vi "Begin.vi"(8 "error in":errorcluster) -> (0 "error out":errorcluster)   [LabVIEW 2019]
doc: "Called before other user functions, this VI is expected to open initial I/O refnums, load in file data, and do all program initialization. Notice that the <B>error out</B> terminal is simply used for data flow. Wiring it to other structures or subVIs ensures that this VI runs first."
uses:
  <vilib>/Rock Robotics/WPI/SafetyOutput/WPI_SafetyOutputConfigMenu.ctl
  <vilib>/Rock Robotics/WPI/DriverStation/WPI_DriverStationRobotMode2.ctl
  <vilib>/Rock Robotics/WPI/Joystick/WPI_JoystickDeviceEnum.ctl
  <vilib>/Rock Robotics/WPI/ThirdParty/REV Robotics/SPARK MAX/Typedef/Spark MAX Idle Mode.ctl
  <vilib>/Rock Robotics/WPI/ThirdParty/REV Robotics/SPARK MAX/Typedef/Spark MAX Motor Type.ctl
  <vilib>/Rock Robotics/WPI/Solenoid/WPI_SolenoidChannel.ctl
  <vilib>/Rock Robotics/WPI/ThirdParty/Phoenix-LabVIEW/Motor Controller/Controls/CTRE_Phoenix_MotorControl_ControlMode.ctl
  <vilib>/Rock Robotics/SystemInterfaces/DIO/FPGA_DIOChannel.ctl
  <vilib>/Rock Robotics/WPI/Encoder/WPI_EncoderType.ctl
  Robot Global Data.vi
  <vilib>/Rock Robotics/Network Tables/NT Write String Array.vi
  <vilib>/Rock Robotics/WPI/RobotDrive/WPI_RobotDriveOpen2MotorWithExistingMotors.vi
  <vilib>/Rock Robotics/WPI/Solenoid/WPI_SolenoidOpenDouble.vi
  <vilib>/Rock Robotics/WPI/Counter/WPI_CounterDigitalInputToDigitalSource.vi
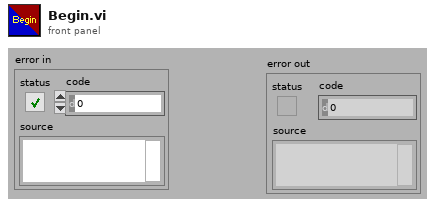
[diagram p1: front panel]
types:
  T1 = typedef "WPI_EncoderType.ctl" = enum16{"1x", "2x", "4x"}
  T2 = typedef "FPGA_DIOChannel.ctl" = enum8{"DIO 0", "DIO 1", "DIO 2", "DIO 3", "DIO 4", "DIO 5", "DIO 6", "DIO 7", "DIO 8", "DIO 9", "DIO MXP 0", "DIO MXP 1", "DIO MXP 2", "DIO MXP 3", "DIO MXP 4", "DIO MXP 5", "DIO MXP 6", "DIO MXP 7", "DIO MXP 8", "DIO MXP 9", "DIO MXP 10", "DIO MXP 11", "DIO MXP 12", "DIO MXP 13", "DIO MXP 14", "DIO MXP 15", "SPI Port CS1", "SPI Port CS2", "SPI Port CS3", "SPI Port MISO", "SPI Port MOSI", "Invalid"}
  T3 = typedef "CTRE_Phoenix_MotorControl_ControlMode.ctl" = u16
  T4 = typedef "WPI_SolenoidChannel.ctl" = enum8{"Solenoid 0", "Solenoid 1", "Solenoid 2", "Solenoid 3", "Solenoid 4", "Solenoid 5", "Solenoid 6", "Solenoid 7", "Invalid"}
  T5 = typedef "WPI_JoystickDeviceEnum.ctl" = enum16{"USB 0", "USB 1", "USB 2", "USB 3", "USB 4", "USB 5"}
  T6 = typedef "Spark MAX Motor Type.ctl" = enum16{"Brushed", "Brushless"}
  T7 = typedef "Spark MAX Idle Mode.ctl" = enum16{"Coast", "Brake"}
  T8 = typedef "WPI_DriverStationRobotMode2.ctl" = enum16{"Autonomous Disabled", "Autonomous Enabled", "Teleop Disabled", "Teleop Enabled", "Disconnected", "Finish", "Test Disabled", "Test Enabled", "Emergency Stopped"}
  T9 = typedef "WPI_SafetyOutputConfigMenu.ctl" = enum16{"Enable", "Disable"}
  T10 = typedef "WPI_MotorControlDeviceRef.ctl" = cluster{"DeviceStatus":errorcluster, "Type":T11, "PWM":cluster{"PWM Channel":T12, "DeadBand":T13}, "CAN":cluster{"Device Number":u8, "SetOutput VI Ref":variant, "GetOutput VI Ref":variant, "Enable VI Ref":variant, "Disable VI Ref":variant, "Data":variant}, "Invert":bool, "DIO PWM":cluster{"PWM \"Enable\" Channel":T12, "DIOChannel":T2, "PWM Rate":dbl}}
  T11 = typedef "WPI_MotorControlType.ctl" = enum16{"PWM", "CAN", "DIO PWM"}
  T12 = typedef "FPGA_DIOPWMChannel.ctl" = enum8{"PWM 0", "PWM 1", "PWM 2", "PWM 3", "PWM 4", "PWM 5", "PWM 6", "PWM 7", "PWM 8", "PWM 9", "PWM MXP 0", "PWM MXP 1", "PWM MXP 2", "PWM MXP 3", "PWM MXP 4", "PWM MXP 5", "PWM MXP 6", "PWM MXP 7", "PWM MXP 8", "PWM MXP 9", "Invalid"}
  T13 = typedef "WPI_PWMDeadband.ctl" = cluster{"Name":string, "maxPositivePwm":i32, "minPositivePwm":i32, "centerPwm":i32, "maxNegativePwm":i32, "minNegativePwm":i32, "angularRange":u16}
  T14 = typedef "WPI_RobotDriveDevRef.ctl" = cluster{"DevStatus":errorcluster, "Motors[]":T10[], "Square Inputs":bool, "Max Output":dbl}
  T15 = typedef "WPI_JoystickDevRef.ctl" = cluster{"Device":T5}
  T16 = typedef "WPI_SolenoidDevRef.ctl" = cluster{"DevStatus":errorcluster, "Pneumatics Control Module":u8, "Forward Solenoid Channel":T4, "Reverse Solenoid Channel":T4}
  T17 = typedef "WPI_DigitalInputDevRef.ctl" = cluster{"DevStatus":errorcluster, "DIO Channel":T2}
  T18 = typedef "FPGA_CounterEncoderSourceConvertionLVSourceType.ctl" = cluster{"DevStatus":errorcluster, "AnalogTriggerMode?":bool, "DigitalMode":cluster{"DIO Channel":T19}, "AnalogTriggerMode":cluster{"AnalogTriggerIndex":T20, "OutputType":T21}}
  T19 = typedef "FPGA_DIODigitalSourceChannel.ctl" = enum8{"DIO 0", "DIO 1", "DIO 2", "DIO 3", "DIO 4", "DIO 5", "DIO 6", "DIO 7", "DIO 8", "DIO 9", "DIO MXP 0", "DIO MXP 1", "DIO MXP 2", "DIO MXP 3", "DIO MXP 4", "DIO MXP 5", "DIO MXP 6", "DIO MXP 7", "DIO MXP 8", "DIO MXP 9", "DIO MXP 10", "DIO MXP 11", "DIO MXP 12", "DIO MXP 13", "DIO MXP 14", "DIO MXP 15", "SPI Port CS1", "SPI Port CS2", "SPI Port CS3", "SPI Port MISO", "SPI Port MOSI", "Disabled"}
  T20 = typedef "FPGA_AnalogTriggerIndex.ctl" = enum8{"Trig 0", "Trig 1", "Trig 2", "Trig 3", "Trig 4", "Trig 5", "Trig 6", "Trig 7", "Invalid"}
  T21 = typedef "FPGA_AnalogTriggerOutType.ctl" = enum16{"InWindow", "TriggerState", "Rising", "Falling"}
  T22 = typedef "WPI_EncoderDevRef.ctl" = cluster{"DevStatus":errorcluster, "EncoderIndex":T23, "CounterIndex":T24, "DistancePerCount":dbl, "Decoding Type":T1}
  T23 = typedef "FPGA_EncoderIdx.ctl" = enum8{"Enc 0", "Enc 1", "Enc 2", "Enc 3", "Enc 4", "Enc 5", "Enc 6", "Enc 7", "Invalid"}
  T24 = typedef "FPGA_CounterCtrSystemIndex.ctl" = enum8{"Ctr 0", "Ctr 1", "Ctr 2", "Ctr 3", "Ctr 4", "Ctr 5", "Ctr 6", "Ctr 7", "Invalid"}
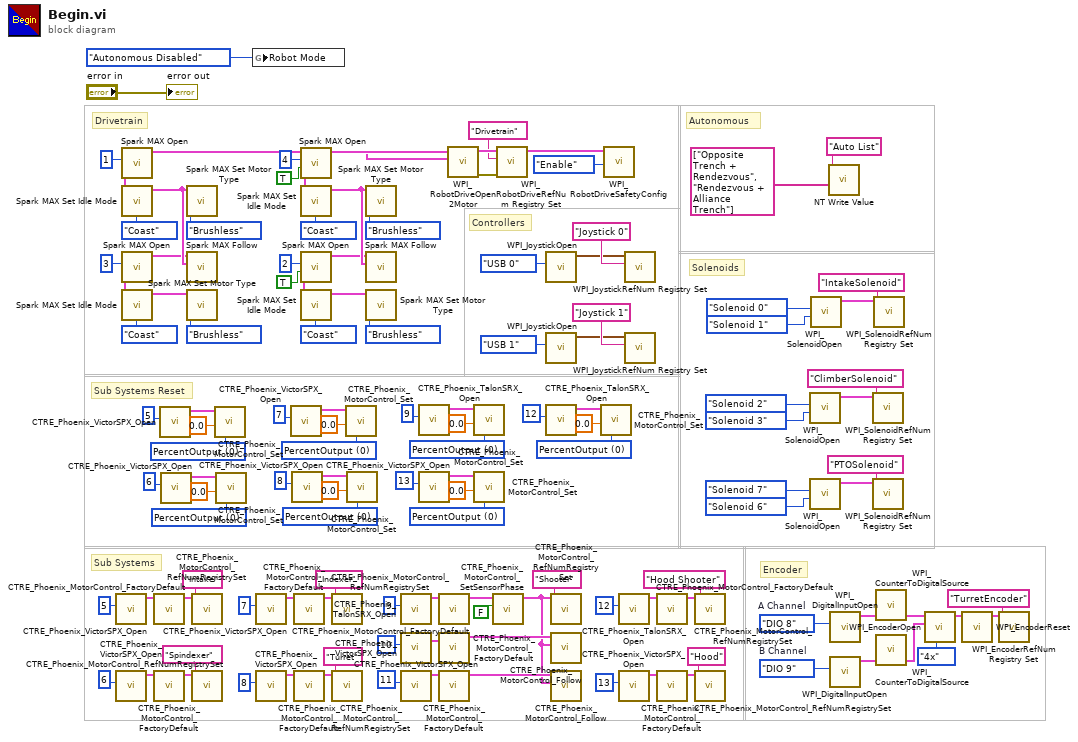
[diagram p0: block diagram]
diagram:
  w8 = FPGA_DIOChannel."DIO 9"  # B Channel
  w7 = FPGA_DIOChannel."DIO 8"  # A Channel
  w16 = T3 0 items=["PercentOutput"=0, "Position"=1, "Velocity"=2, "Current"=3, "Follower"=5, "MotionProfile"=6, "MotionMagic"=7, "MotionProfileArc"=10, "Disabled"=15] ("Control Mode")
  w19 = T3 0 items=["PercentOutput"=0, "Position"=1, "Velocity"=2, "Current"=3, "Follower"=5, "MotionProfile"=6, "MotionMagic"=7, "MotionProfileArc"=10, "Disabled"=15] ("Control Mode")
  w24 = T3 0 items=["PercentOutput"=0, "Position"=1, "Velocity"=2, "Current"=3, "Follower"=5, "MotionProfile"=6, "MotionMagic"=7, "MotionProfileArc"=10, "Disabled"=15] ("Control Mode")
  w32 = T3 0 items=["PercentOutput"=0, "Position"=1, "Velocity"=2, "Current"=3, "Follower"=5, "MotionProfile"=6, "MotionMagic"=7, "MotionProfileArc"=10, "Disabled"=15] ("Control Mode")
  w29 = T3 0 items=["PercentOutput"=0, "Position"=1, "Velocity"=2, "Current"=3, "Follower"=5, "MotionProfile"=6, "MotionMagic"=7, "MotionProfileArc"=10, "Disabled"=15] ("Control Mode")
  w37 = T3 0 items=["PercentOutput"=0, "Position"=1, "Velocity"=2, "Current"=3, "Follower"=5, "MotionProfile"=6, "MotionMagic"=7, "MotionProfileArc"=10, "Disabled"=15] ("Control Mode")
  w39 = T3 0 items=["PercentOutput"=0, "Position"=1, "Velocity"=2, "Current"=3, "Follower"=5, "MotionProfile"=6, "MotionMagic"=7, "MotionProfileArc"=10, "Disabled"=15] ("Control Mode")
  # "Encoder"
  # "Autonomous"
  # "Sub Systems Reset"
  # "Solenoids"
  # "Controllers"
  # "Sub Systems"
  # "Drivetrain"
  n1 = call <vilib>:"CTRE_Phoenix_VictorSPX_Open.vi"("Device Number"=u8 5) -> ("CAN Talon SRX Ref"=w62:T10)  [unwired: 9 in, 1 out]
  n2 = call <vilib>:"CTRE_Phoenix_VictorSPX_Open.vi"("Device Number"=u8 6) -> ("CAN Talon SRX Ref"=w64:T10)  [unwired: 9 in, 1 out]
  n3 = call <vilib>:"Spark MAX Open.vi"("Device Number"=u8 1) -> ("MotorControlDeviceRef"=w88:T10)  [unwired: 9 in, 1 out]
  n4 = call <vilib>:"Spark MAX Set Idle Mode.vi"("Idle Mode"=Spark_MAX_Idle_Mode."Coast", "MotorControlDeviceRef in"=w88) -> ("MotorControlDeviceRef out"=w104:T10)  [unwired: 8 in, 1 out]
  n5 = call <vilib>:"Spark MAX Open.vi"("Device Number"=u8 3) -> ("MotorControlDeviceRef"=w103:T10)  [unwired: 9 in, 1 out]
  n6 = call <vilib>:"Spark MAX Set Idle Mode.vi"("Idle Mode"=Spark_MAX_Idle_Mode."Coast", "MotorControlDeviceRef in"=w103) -> ("MotorControlDeviceRef out"=w108:T10)  [unwired: 8 in, 1 out]
  n7 = call <vilib>:"CTRE_Phoenix_MotorControl_FactoryDefault.vi"("PhoenixMotorControlDevRef"=w62) -> ("PhoenixMotorControlDevRef"=w63:T10)  [unwired: 9 in, 1 out]
  n8 = call <vilib>:"CTRE_Phoenix_MotorControl_FactoryDefault.vi"("PhoenixMotorControlDevRef"=w64) -> ("PhoenixMotorControlDevRef"=w65:T10)  [unwired: 9 in, 1 out]
  n9 = call <vilib>:"CTRE_Phoenix_VictorSPX_Open.vi"("Device Number"=u8 5) -> ("CAN Talon SRX Ref"=w36:T10)  [unwired: 9 in, 1 out]
  n10 = call <vilib>:"CTRE_Phoenix_VictorSPX_Open.vi"("Device Number"=u8 6) -> ("CAN Talon SRX Ref"=w40:T10)  [unwired: 9 in, 1 out]
  n11 = call <vilib>:"Spark MAX Set Motor Type.vi"("Motor Type"=Spark_MAX_Motor_Type."Brushless", "MotorControlDevRef"=w104) -> ()  [unwired: 8 in, 2 out]
  n12 = call <vilib>:"Spark MAX Follow.vi"("Master Controller"=w104, "MotorControlDeviceRef"=w103) -> ()  [unwired: 8 in, 2 out]
  n13 = call <vilib>:"Spark MAX Set Motor Type.vi"("Motor Type"=Spark_MAX_Motor_Type."Brushless", "MotorControlDevRef"=w108) -> ()  [unwired: 8 in, 2 out]
  n14 = call <vilib>:"CTRE_Phoenix_MotorControl_RefNumRegistrySet.vi"("refnum name"="Intake", "PhoenixMotorControlDevRef"=w63) -> ()  [unwired: 8 in, 2 out]
  n15 = call <vilib>:"CTRE_Phoenix_MotorControl_RefNumRegistrySet.vi"("refnum name"="Spindexer", "PhoenixMotorControlDevRef"=w65) -> ()  [unwired: 8 in, 2 out]
  n16 = call <vilib>:"CTRE_Phoenix_MotorControl_Set.vi"("Output"=0.0, "Control Mode"=w37, "PhoenixMotorControlDevRef"=w36) -> ()  [unwired: 7 in, 2 out]
  n17 = call <vilib>:"CTRE_Phoenix_MotorControl_Set.vi"("Output"=0.0, "Control Mode"=w39, "PhoenixMotorControlDevRef"=w40) -> ()  [unwired: 7 in, 2 out]
  n18 = global write "Robot Global Data.vi" "Robot Mode"(WPI_DriverStationRobotMode2."Autonomous Disabled" ("Robot Mode")) -> ()
  n19 = call <vilib>:"CTRE_Phoenix_VictorSPX_Open.vi"("Device Number"=u8 7) -> ("CAN Talon SRX Ref"=w58:T10)  [unwired: 9 in, 1 out]
  n20 = call <vilib>:"CTRE_Phoenix_VictorSPX_Open.vi"("Device Number"=u8 8) -> ("CAN Talon SRX Ref"=w54:T10)  [unwired: 9 in, 1 out]
  n21 = call <vilib>:"CTRE_Phoenix_VictorSPX_Open.vi"("Device Number"=u8 7) -> ("CAN Talon SRX Ref"=w33:T10)  [unwired: 9 in, 1 out]
  n22 = call <vilib>:"CTRE_Phoenix_VictorSPX_Open.vi"("Device Number"=u8 8) -> ("CAN Talon SRX Ref"=w28:T10)  [unwired: 9 in, 1 out]
  n23 = call <vilib>:"CTRE_Phoenix_MotorControl_FactoryDefault.vi"("PhoenixMotorControlDevRef"=w58) -> ("PhoenixMotorControlDevRef"=w59:T10)  [unwired: 9 in, 1 out]
  n24 = call <vilib>:"CTRE_Phoenix_MotorControl_FactoryDefault.vi"("PhoenixMotorControlDevRef"=w54) -> ("PhoenixMotorControlDevRef"=w55:T10)  [unwired: 9 in, 1 out]
  n25 = call <vilib>:"Spark MAX Open.vi"("Invert"=TRUE, "Device Number"=u8 4) -> ("MotorControlDeviceRef"=w87:T10)  [unwired: 8 in, 1 out]
  n26 = call <vilib>:"Spark MAX Set Idle Mode.vi"("Idle Mode"=Spark_MAX_Idle_Mode."Coast", "MotorControlDeviceRef in"=w87) -> ("MotorControlDeviceRef out"=w95:T10)  [unwired: 8 in, 1 out]
  n27 = call <vilib>:"Spark MAX Open.vi"("Invert"=TRUE, "Device Number"=u8 2) -> ("MotorControlDeviceRef"=w94:T10)  [unwired: 8 in, 1 out]
  n28 = call <vilib>:"Spark MAX Set Idle Mode.vi"("Idle Mode"=Spark_MAX_Idle_Mode."Coast", "MotorControlDeviceRef in"=w94) -> ("MotorControlDeviceRef out"=w99:T10)  [unwired: 8 in, 1 out]
  n29 = call <vilib>:"CTRE_Phoenix_MotorControl_RefNumRegistrySet.vi"("refnum name"="Indexer", "PhoenixMotorControlDevRef"=w59) -> ()  [unwired: 8 in, 2 out]
  n30 = call <vilib>:"CTRE_Phoenix_MotorControl_RefNumRegistrySet.vi"("refnum name"="Turret", "PhoenixMotorControlDevRef"=w55) -> ()  [unwired: 8 in, 2 out]
  n31 = call <vilib>:"CTRE_Phoenix_MotorControl_Set.vi"("Output"=0.0, "Control Mode"=w32, "PhoenixMotorControlDevRef"=w33) -> ()  [unwired: 7 in, 2 out]
  n32 = call <vilib>:"CTRE_Phoenix_MotorControl_Set.vi"("Output"=0.0, "Control Mode"=w29, "PhoenixMotorControlDevRef"=w28) -> ()  [unwired: 7 in, 2 out]
  n33 = call <vilib>:"Spark MAX Set Motor Type.vi"("Motor Type"=Spark_MAX_Motor_Type."Brushless", "MotorControlDevRef"=w95) -> ()  [unwired: 8 in, 2 out]
  n34 = call <vilib>:"Spark MAX Follow.vi"("Master Controller"=w95, "MotorControlDeviceRef"=w94) -> ()  [unwired: 8 in, 2 out]
  n35 = call <vilib>:"Spark MAX Set Motor Type.vi"("Motor Type"=Spark_MAX_Motor_Type."Brushless", "MotorControlDevRef"=w99) -> ()  [unwired: 8 in, 2 out]
  n36 = call <vilib>:"CTRE_Phoenix_TalonSRX_Open.vi"("Device Number"=u8 9) -> ("CAN Talon SRX Ref"=w53:T10)  [unwired: 9 in, 1 out]
  n37 = call <vilib>:"CTRE_Phoenix_VictorSPX_Open.vi"("Device Number"=u8 10) -> ("CAN Talon SRX Ref"=w52:T10)  [unwired: 9 in, 1 out]
  n38 = call <vilib>:"CTRE_Phoenix_VictorSPX_Open.vi"("Device Number"=u8 11) -> ("CAN Talon SRX Ref"=w51:T10)  [unwired: 9 in, 1 out]
  n39 = call <vilib>:"CTRE_Phoenix_TalonSRX_Open.vi"("Device Number"=u8 9) -> ("CAN Talon SRX Ref"=w20:T10)  [unwired: 9 in, 1 out]
  n40 = call <vilib>:"CTRE_Phoenix_VictorSPX_Open.vi"("Device Number"=u8 13) -> ("CAN Talon SRX Ref"=w23:T10)  [unwired: 9 in, 1 out]
  n41 = call <vilib>:"CTRE_Phoenix_MotorControl_FactoryDefault.vi"("PhoenixMotorControlDevRef"=w53) -> ("PhoenixMotorControlDevRef"=w13:T10)  [unwired: 9 in, 1 out]
  n42 = call <vilib>:"CTRE_Phoenix_MotorControl_FactoryDefault.vi"("PhoenixMotorControlDevRef"=w52) -> ("PhoenixMotorControlDevRef"=w49:T10)  [unwired: 9 in, 1 out]
  n43 = call <vilib>:"CTRE_Phoenix_MotorControl_FactoryDefault.vi"("PhoenixMotorControlDevRef"=w51) -> ("PhoenixMotorControlDevRef"=w50:T10)  [unwired: 9 in, 1 out]
  n44 = call-poly <vilib>:"WPI_RobotDriveOpen2Motor.vi"("Right Motor Dev Ref"=w87, "Left Motor Dev Ref"=w88) -> ("error out"=w121:errorcluster, "RobotDriveDevRef"=w123:T14)  [unwired: 3 in, 5 out]
  n45 = call <vilib>:"CTRE_Phoenix_MotorControl_Set.vi"("Output"=0.0, "Control Mode"=w19, "PhoenixMotorControlDevRef"=w20) -> ()  [unwired: 7 in, 2 out]
  n46 = call <vilib>:"CTRE_Phoenix_MotorControl_Set.vi"("Output"=0.0, "Control Mode"=w24, "PhoenixMotorControlDevRef"=w23) -> ()  [unwired: 7 in, 2 out]
  n47 = call <vilib>:"CTRE_Phoenix_MotorControl_SetSensorPhase.vi"("PhaseSensor"=FALSE, "PhoenixMotorControlDevRef"=w13) -> ("PhoenixMotorControlDevRef"=w11:T10)  [unwired: 8 in, 1 out]
  n48 = call <vilib>:"WPI_RobotDriveRefNum Registry Set.vi"("error in (no error)"=w121, "refnum name"="Drivetrain", "RobotDriveDevRef"=w123) -> ("RobotDriveDevRef"=w120:T14)  [unwired: 1 in, 7 out]
  n49 = call <vilib>:"WPI_JoystickOpen.vi"("JoystickDevice"=WPI_JoystickDeviceEnum."USB 0") -> ("JoystickDevRef"=w116:T15)  [unwired: 10 in]
  n50 = call <vilib>:"WPI_JoystickOpen.vi"("JoystickDevice"=WPI_JoystickDeviceEnum."USB 1") -> ("JoystickDevRef"=w90:T15)  [unwired: 10 in]
  n51 = call <vilib>:"CTRE_Phoenix_TalonSRX_Open.vi"("Device Number"=u8 12) -> ("CAN Talon SRX Ref"=w15:T10)  [unwired: 9 in, 1 out]
  n52 = call <vilib>:"CTRE_Phoenix_MotorControl_RefNumRegistrySet.vi"("refnum name"="Shooter", "PhoenixMotorControlDevRef"=w11) -> ()  [unwired: 8 in, 2 out]
  n53 = call <vilib>:"CTRE_Phoenix_MotorControl_Follow.vi"("Master Controller to Follow"=w11, "PhoenixMotorControlDevRef"=w49) -> ()  [unwired: 8 in, 2 out]
  n54 = call <vilib>:"CTRE_Phoenix_MotorControl_Follow.vi"("Master Controller to Follow"=w11, "PhoenixMotorControlDevRef"=w50) -> ()  [unwired: 8 in, 2 out]
  n55 = call <vilib>:"CTRE_Phoenix_MotorControl_Set.vi"("Output"=0.0, "Control Mode"=w16, "PhoenixMotorControlDevRef"=w15) -> ()  [unwired: 7 in, 2 out]
  n56 = call <vilib>:"WPI_RobotDriveSafetyConfig.vi"("mode"=WPI_SafetyOutputConfigMenu."Enable", "RobotDriveDevRef"=w120) -> ()  [unwired: 8 in, 2 out]
  n57 = call <vilib>:"CTRE_Phoenix_TalonSRX_Open.vi"("Device Number"=u8 12) -> ("CAN Talon SRX Ref"=w46:T10)  [unwired: 9 in, 1 out]
  n58 = call <vilib>:"CTRE_Phoenix_VictorSPX_Open.vi"("Device Number"=u8 13) -> ("CAN Talon SRX Ref"=w41:T10)  [unwired: 9 in, 1 out]
  n59 = call <vilib>:"WPI_JoystickRefNum Registry Set.vi"("refnum name"="Joystick 0", "JoystickDevRef"=w116) -> ()  [unwired: 8 in, 2 out]
  n60 = call <vilib>:"WPI_JoystickRefNum Registry Set.vi"("refnum name"="Joystick 1", "JoystickDevRef"=w90) -> ()  [unwired: 8 in, 2 out]
  n61 = call <vilib>:"CTRE_Phoenix_MotorControl_FactoryDefault.vi"("PhoenixMotorControlDevRef"=w46) -> ("PhoenixMotorControlDevRef"=w47:T10)  [unwired: 9 in, 1 out]
  n62 = call <vilib>:"CTRE_Phoenix_MotorControl_FactoryDefault.vi"("PhoenixMotorControlDevRef"=w41) -> ("PhoenixMotorControlDevRef"=w42:T10)  [unwired: 9 in, 1 out]
  n63 = call <vilib>:"CTRE_Phoenix_MotorControl_RefNumRegistrySet.vi"("refnum name"="Hood Shooter", "PhoenixMotorControlDevRef"=w47) -> ()  [unwired: 8 in, 2 out]
  n64 = call <vilib>:"CTRE_Phoenix_MotorControl_RefNumRegistrySet.vi"("refnum name"="Hood", "PhoenixMotorControlDevRef"=w42) -> ()  [unwired: 8 in, 2 out]
  n65 = call-poly <vilib>:"WPI_SolenoidOpen.vi"("Reverse Solenoid Channel"=WPI_SolenoidChannel."Solenoid 3", "Forward Solenoid Channel"=WPI_SolenoidChannel."Solenoid 2") -> ("SolenoidDevRef"=w74:T16)  [unwired: 8 in, 1 out]
  n66 = call-poly <vilib>:"WPI_SolenoidOpen.vi"("Reverse Solenoid Channel"=WPI_SolenoidChannel."Solenoid 6", "Forward Solenoid Channel"=WPI_SolenoidChannel."Solenoid 7") -> ("SolenoidDevRef"=w70:T16)  [unwired: 8 in, 1 out]
  n67 = call-poly <vilib>:"WPI_SolenoidOpen.vi"("Reverse Solenoid Channel"=WPI_SolenoidChannel."Solenoid 1", "Forward Solenoid Channel"=WPI_SolenoidChannel."Solenoid 0") -> ("SolenoidDevRef"=w78:T16)  [unwired: 8 in, 1 out]
  n68 = call-poly <vilib>:"NT Write Value.vi"("String Array"=string[] ["Opposite Trench + Rendezvous", "Rendezvous + Alliance Trench"], "Name"="Auto List") -> ()  [unwired: 9 in, 1 out]
  n69 = call <vilib>:"WPI_DigitalInputOpen.vi"("DIO Channel"=w7) -> ("DigitalInputDevRef"=w5:T17)  [unwired: 1 in, 9 out]
  n70 = call <vilib>:"WPI_DigitalInputOpen.vi"("DIO Channel"=w8) -> ("DigitalInputDevRef"=w6:T17)  [unwired: 1 in, 9 out]
  n71 = call <vilib>:"WPI_SolenoidRefNum Registry Set.vi"("refnum name"="ClimberSolenoid", "SolenoidDevRef"=w74) -> ()  [unwired: 8 in, 2 out]
  n72 = call <vilib>:"WPI_SolenoidRefNum Registry Set.vi"("refnum name"="PTOSolenoid", "SolenoidDevRef"=w70) -> ()  [unwired: 8 in, 2 out]
  n73 = call <vilib>:"WPI_SolenoidRefNum Registry Set.vi"("refnum name"="IntakeSolenoid", "SolenoidDevRef"=w78) -> ()  [unwired: 8 in, 2 out]
  n74 = call-poly <vilib>:"WPI_CounterToDigitalSource.vi"("DigitalInputDevRef"=w5) -> ("Digital Source"=w9:T18)  [unwired: 6 out]
  n75 = call-poly <vilib>:"WPI_CounterToDigitalSource.vi"("DigitalInputDevRef"=w6) -> ("Digital Source"=w10:T18)  [unwired: 6 out]
  n76 = call <vilib>:"WPI_EncoderOpen.vi"("Decoding Type"=WPI_EncoderType."4x", "BSource"=w10, "ASource"=w9) -> ("EncoderDevRef"=w3:T22)  [unwired: 7 in, 1 out]
  n77 = call <vilib>:"WPI_EncoderReset.vi"("EncoderDevRef"=w3) -> ("EncoderDevRef"=w2:T22)  [unwired: 9 in, 1 out]
  n78 = call <vilib>:"WPI_EncoderRefNum Registry Set.vi"("refnum name"="TurretEncoder", "EncoderDevRef"=w2) -> ()  [unwired: 8 in, 2 out]
  "error out" <- "error in"
